vi "Radius Search Int.vi"(0 "KD Tree Int in":refnum<class "KD Tree Int.lvclass">, 1 "Radius":sgl=1.0, 3 "Max Neighbors":i32=1, 5 "Points":i32[][](array[numeric]), 11 "error in (no error)":errorcluster) -> (4 "KD Tree Int out":refnum<class "KD Tree Int.lvclass">, 6 "Indices":i32[][](array[numeric]), 8 "Dists":sgl[][](array[numeric]), 10 "N Found":i32[](array[numeric]), 15 "error out":errorcluster)   [LabVIEW 2020, in "KD Tree.lvlib" / "KD Tree Int.lvclass"]
uses:
  KD Tree Int.lvclass
  E:/Labview/LV 2020/Libs/flann/flann/Classes/KD Tree/KD Tree.lvclass
  KD Tree/KD Tree.lvclass/KD Tree.ctl
  KD Tree/Read index_ptr.vi
  KD Tree/Read flann_params.vi
  KD Tree Int.lvclass/KD Tree Int.ctl
  KD Tree.lvlib
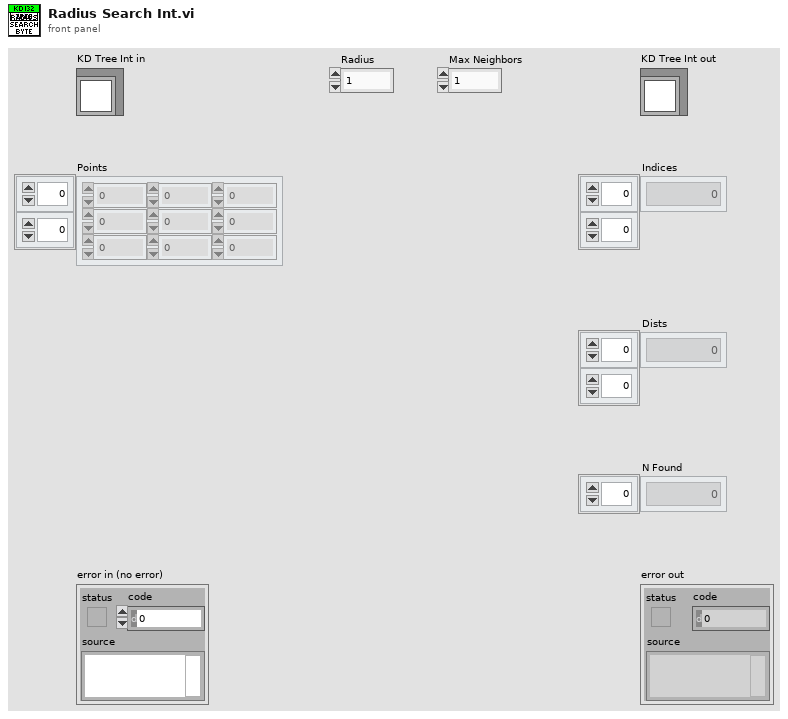
[diagram p1: front panel]
types:
  T1 = typedef "KD Tree.lvlib/Distance Type.ctl" = u32
  T2 = typedef "KD Tree.lvlib/Flann Params.ctl" = cluster{"algorithm":u32, "checks":i32, "eps":sgl, "sorted":i32, "max_neighbors":i32, "cores":i32, "trees":i32, "leaf_max_size":i32, "branching":i32, "iterations":i32, "centers_init":u32, "cb_index":sgl, "target_precision":sgl, "build_weight":sgl, "memory_weight":sgl, "sample_fraction":sgl, "table_number_":u32, "key_size_":u32, "multi_probe_level_":u32, "log_level":u32, "random_seed":i32}
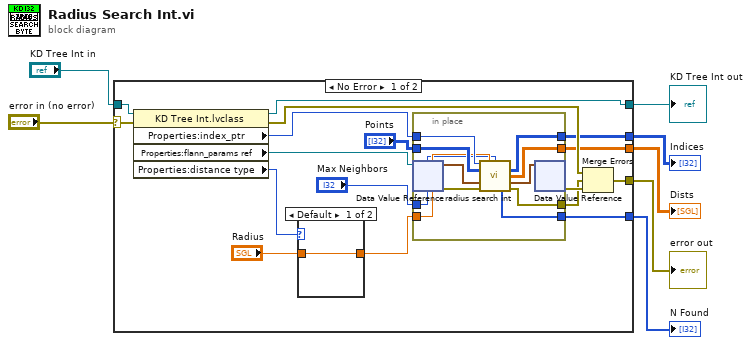
[diagram p0: block diagram]
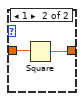
[diagram p2: hidden frame]
diagram:
  n1 = case shown="No Error" "error in (no error)" {
    selector: "error in (no error)" -> [w24 w40]
    tunnel: [w18 w40] -> w4
    tunnel: [w22 w39] -> w5
    tunnel: "KD Tree Int in" -> [w23 w39]
    tunnel: [w10 _] -> w3
    tunnel: [w9 _] -> w2
    tunnel: [w8 _] -> w1
    frame No Error {
      n2 = property class="KD Tree Int.lvclass"(reference=w23, error in=w24) -> (reference out=w22:refnum<class "KD Tree Int.lvclass">, error out=w14:errorcluster, "Properties:index_ptr"=w21:u64, "Properties:flann_params ref"=w19:refnum<data-value>, "Properties:distance type"=w11:T1)
      n3 = case shown="Default" w11 {
        tunnel: "Radius" -> [w25 w27]
        tunnel: [w25 w26] -> w12
        frame Default {
        }
        frame 1 {
          n4 = Square(x=w27) -> (x^2=w26:sgl)
        }
      }
      n5 = in-place {
        in-place-border: w21 -> [w38]
        in-place-border: "Points" -> [w37]
        in-place-border: [w35] -> w9
        in-place-border: [w34] -> w10
        in-place-border: w12 -> [w33]
        in-place-border: "Max Neighbors" -> [w32]
        in-place-border: [w31] -> w8
        in-place-border: [w30] -> w15
        n6 = in-place-dvr #1(w19) -> (w28:T2, w29:errorcluster)
        n7 = call "radius search int.vi"("index_ptr"=w38, "radius"=w33, "max_nn"=w32, "query points"=w37, "flann_params"=w28, "error in (no error)"=w29) -> ("indices out"=w34:i32[][], "dists out"=w35:sgl[][], "flann_params"=w36:T2, "N Found"=w31:i32[], "error out"=w30:errorcluster)  [unwired: 4 in, 1 out]
        n8 = in-place-dvr #1(w36) -> (w17:errorcluster)  [unwired: 1 out]
      }
      n9 = Merge Errors(w14, w15, w17) -> (w18:errorcluster)
    }
    frame Error {
    }
  }
  "error out" <- w4
  "KD Tree Int out" <- w5
  "Indices" <- w3
  "Dists" <- w2
  "N Found" <- w1
